vi "Read XML HW Configuration File_Parse Channels_Tx Channels Detect ID Mismatch.vi"(7 "Label":i32, 8 "error in (no error)":errorcluster, 9 "channel":T1, 10 "messageBuffer ID":i32, 11 "messageBufferIDRef":i32) -> (0 "error out":errorcluster)   [LabVIEW 2017]
uses:
  Controls/Ballard_Channel.ctl
  Controls/Ballard_messageType.ctl
  Controls/Ballard_CWD1.ctl
  Controls/Ballard_minorFrame.ctl
  Controls/Ballard_majorFrame.ctl
  Controls/Ballard_BC.ctl
  Controls/Ballard_RT.ctl
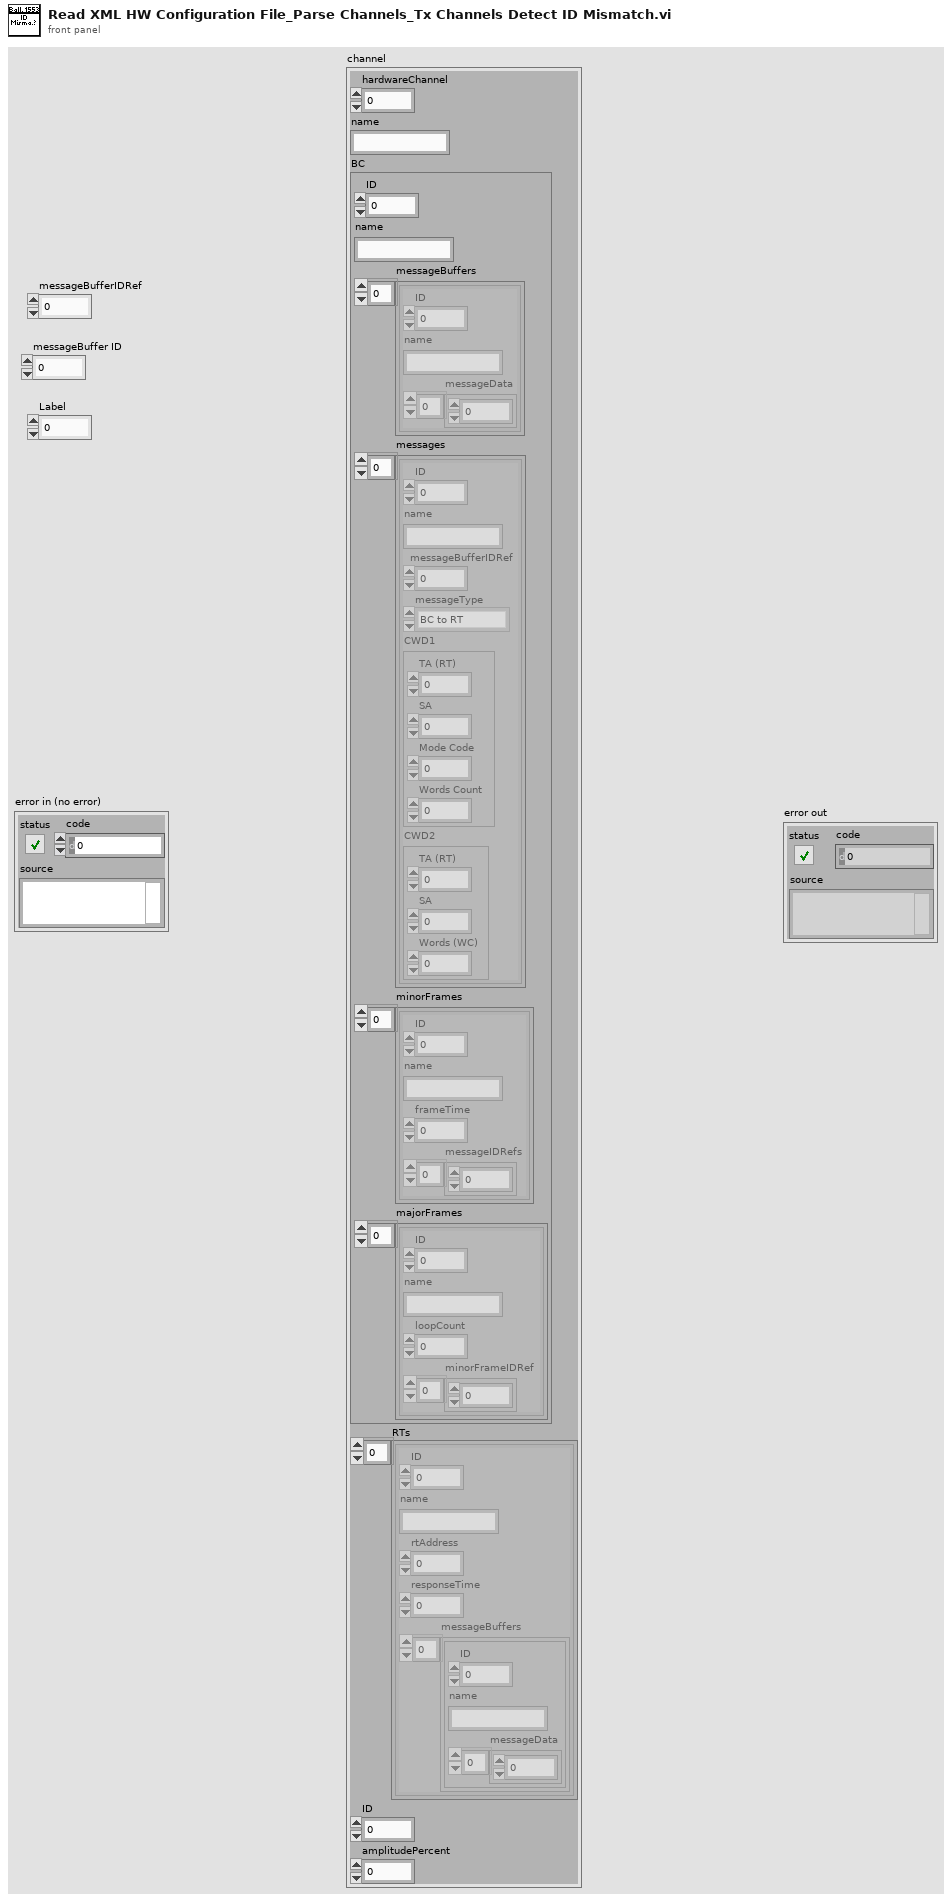
[diagram p1: front panel]
types:
  T1 = typedef "Ballard 1553.lvlib/Ballard_Channel.ctl" = cluster{"hardwareChannel":i32, "name":string, "BC":T2, "RTs":T7[], "ID":i32, "amplitudePercent":dbl}
  T2 = typedef "Ballard 1553.lvlib/Ballard_BC.ctl" = cluster{"ID":i32, "name":string, "messageBuffers":cluster{"ID":i32, "name":string, "messageData":u16[]}[], "messages":cluster{"ID":i32, "name":string, "messageBufferIDRef":i32, "messageType":T3, "CWD1":T4, "CWD2":cluster{"TA (RT)":dbl, "SA":dbl, "Words (WC)":dbl}}[], "minorFrames":T5[], "majorFrames":T6[]}
  T3 = typedef "Ballard 1553.lvlib/Ballard_messageType.ctl" = enum16{"BC to RT", "RT to BC", "RT to RT", "MC (Rx)", "MC (Tx)"}
  T4 = typedef "Ballard 1553.lvlib/Ballard_CWD1.ctl" = cluster{"TA (RT)":i8, "SA":i8, "Mode Code":i8, "Words Count":i8}
  T5 = typedef "Ballard 1553.lvlib/Ballard_minorFrame.ctl" = cluster{"ID":i32, "name":string, "frameTime":i32, "messageIDRefs":i32[]}
  T6 = typedef "Ballard 1553.lvlib/Ballard_majorFrame.ctl" = cluster{"ID":i32, "name":string, "loopCount":i32, "minorFrameIDRef":i32[]}
  T7 = typedef "Ballard 1553.lvlib/Ballard_RT.ctl" = cluster{"ID":i32, "name":string, "rtAddress":i8, "responseTime":i32, "messageBuffers":cluster{"ID":i32, "name":string, "messageData":u16[]}[]}
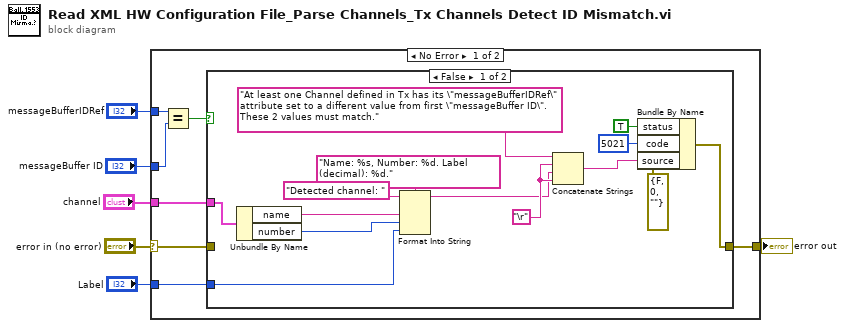
[diagram p0: block diagram]
diagram:
  n1 = case shown="No Error" "error in (no error)" {
    selector: "error in (no error)" -> [w11 w29]
    tunnel: [w10 w29] -> w5
    tunnel: "messageBufferIDRef" -> [w13 _]
    tunnel: "messageBuffer ID" -> [w12 _]
    tunnel: "channel" -> [w9 _]
    tunnel: "Label" -> [w7 _]
    frame No Error {
      n2 = Equal?(x=w13, y=w12) -> (x = y?=w8:bool)
      n3 = case shown="False" w8 {
        tunnel: w11 -> [_ w28]
        tunnel: [w16 w28] -> w10
        tunnel: w9 -> [w15 _]
        tunnel: w7 -> [w14 _]
        frame False {
          w21 = "\r"
          n4 = Unbundle By Name(w15) -> ("name"=w20:string, "number"=w19:u8)
          n5 = Format Into String(format string="Name: %s, Number: %d. Label (decimal): %d.", initial string="Detected channel: ", w20, w19, w14) -> (resulting string=w18:string)  [unwired: 1 in, 1 out]
          n6 = Concatenate Strings("At least one Channel defined in Tx has its \"messageBufferIDRef\" attribute set to a different value from first \"messageBuffer ID\". These 2 values must match.", w21, w18, w21) -> (w24:string)
          n7 = Bundle By Name(cluster=errorcluster {"status"=FALSE, "code"=0, "source"=""} ("error in (no error) 2"), "status"=TRUE, "code"=5021, "source"=w24) -> (w16:errorcluster)
        }
        frame True {
        }
      }
    }
    frame Error {
    }
  }
  "error out" <- w5
